vi "set_instruments (SubVI).vi"(0 "Process list":T5, 1 "Flash lamp settings:":T4={"Output channel (for flashing)"="Dev4/ao0", "Loop iteration"=0, "Path"=path "", "Flash lamp\n settings:"={"Flash lamp?"=FALSE, "Number of cyles\nbetween flashes"=3, "# Pulses"=35, "Stop flashing \nbelow thresh?"=FALSE, "Stop threshold"=0.001, "Pulse voltage?"=FALSE, "Pulse length (ms)"=0.001, "Pulse amp (V)"=0.001}}, 2 "signal type":T1(ring), 4 "electrodes reference":refnum<vi>, 5 "instrument config":T3, 6 "Num samples":i32, 7 "small amp":dbl=1.0 format="%0.2p", 9 "Volt vs pos array":cluster{dbl, dbl}[](array[cluster]), 10 "wfm?":bool, 11 "small amp freq":dbl=10.0 format="%0.2p", 12 "User Def. Wfm Name":string="RANDFREQ", 13 "Add small amp?":bool) -> (14 "Curr threshold":dbl, 18 "DC volts arr":dbl[](array[numeric]), 19 "instrum out":T2)   [LabVIEW 2014]
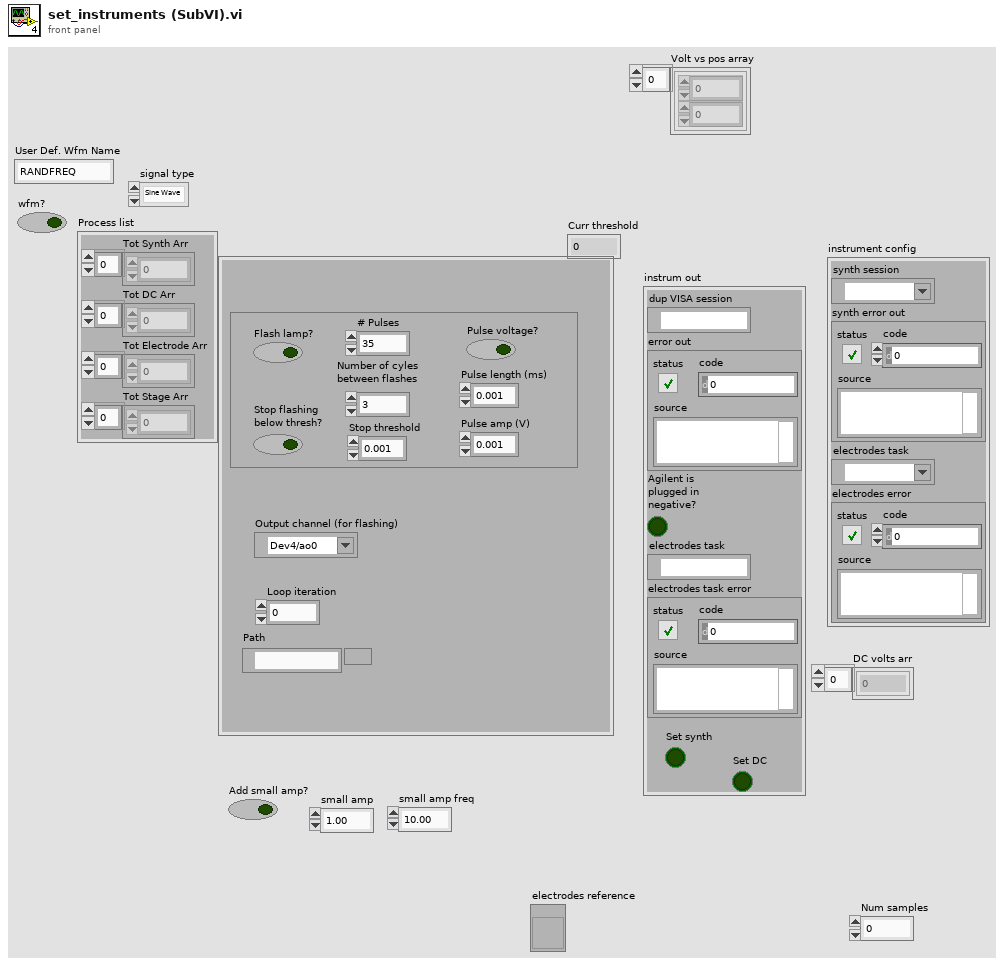
[diagram p1: front panel]
types:
  T1 = enum16{"Sine Wave", "Triangle Wave", "Square Wave", "Sawtooth Wave"}
  T2 = cluster{"dup VISA session":refnum<visa-resource-name>, "error out":errorcluster, "Agilent is \nplugged in \nnegative?":bool, "electrodes task":refnum<k21>, "electrodes task error":errorcluster, "Set synth":bool, "Set DC":bool}
  T3 = cluster{"synth session":refnum<visa-resource-name>, "synth error out":errorcluster, "electrodes task":refnum<k21>, "electrodes error":errorcluster}
  T4 = cluster{"Output channel (for flashing)":tag, "Loop iteration":i32, "Path":path, "Flash lamp\n settings:":cluster{"Flash lamp?":bool, "Number of cyles\nbetween flashes":i32, "# Pulses":i32, "Stop flashing \nbelow thresh?":bool, "Stop threshold":dbl, "Pulse voltage?":bool, "Pulse length (ms)":dbl, "Pulse amp (V)":dbl}}
  T5 = cluster{"Tot Synth Arr":dbl[], "Tot DC Arr":dbl[], "Tot Electrode Arr":dbl[], "Tot Stage Arr":dbl[]}
  T6 = cluster{"Flash lamp?":bool, "Number of cyles\nbetween flashes":i32, "# Pulses":i32, "Stop flashing \nbelow thresh?":bool, "Stop threshold":dbl, "Pulse voltage?":bool, "Pulse length (ms)":dbl, "Pulse amp (V)":dbl}
  T7 = cluster{"dup VISA session":refnum<visa-resource-name>, "error out":errorcluster, "Agilent is \nplugged in \nnegative?":bool, "electrodes task 2":refnum<k21>, "electrodes task error 2":errorcluster, "Set synth?":bool, "Set DC?":bool}
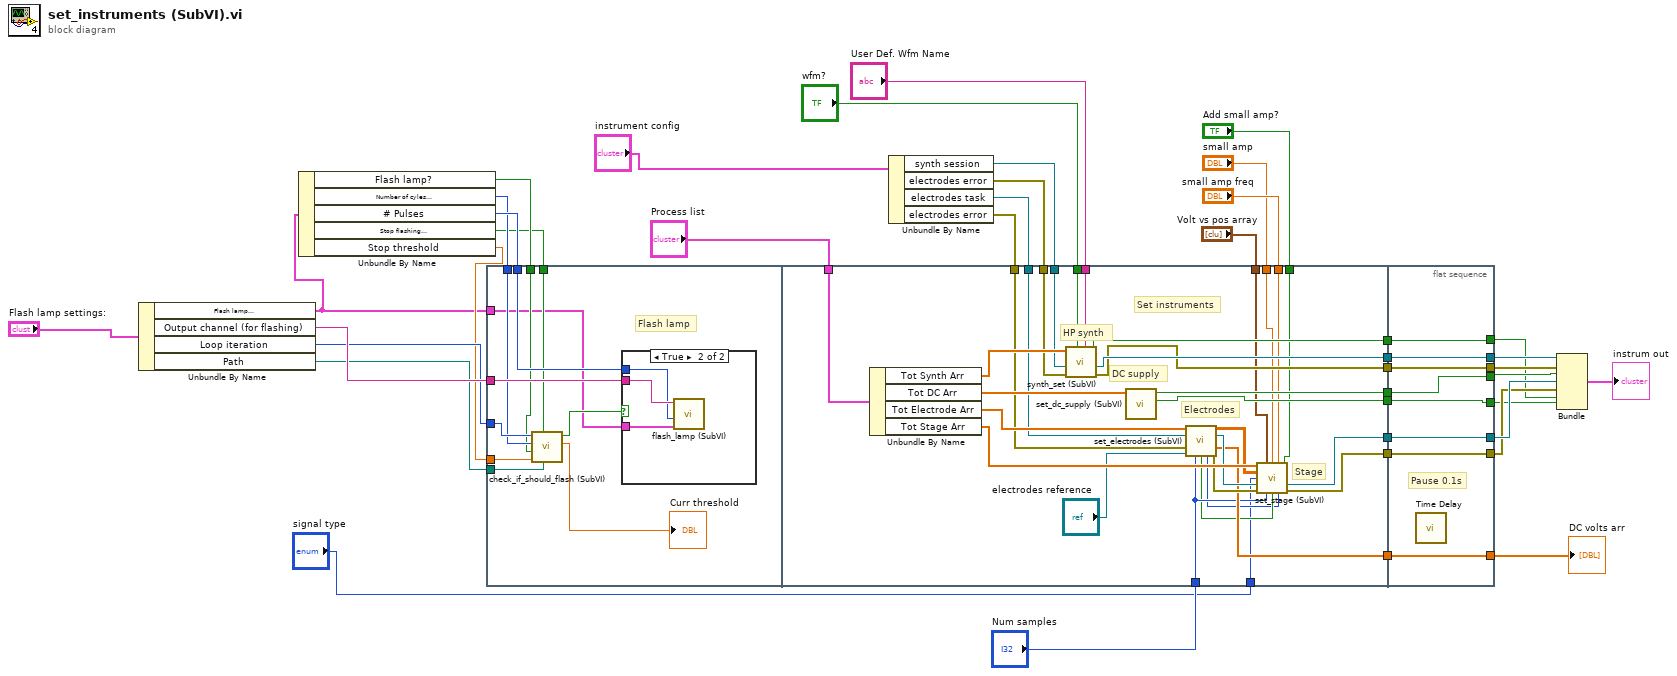
[diagram p0: block diagram]
diagram:
  n1 = Unbundle By Name("Flash lamp settings:") -> ("Flash lamp\n settings:"=w2:T6, "Output channel (for flashing)"=w39:tag, "Loop iteration"=w37:i32, "Path"=w34:path)
  n2 = Unbundle By Name(w2) -> ("Flash lamp?"=w35:bool, "Number of cyles\nbetween flashes"=w36:i32, "# Pulses"=w38:i32, "Stop flashing \nbelow thresh?"=w32:bool, "Stop threshold"=w33:dbl)
  n3 = flat-sequence {
    tunnel: w39 -> [w52]
    tunnel: w38 -> [w51]
    tunnel: w37 -> [w50]
    tunnel: w36 -> [w49]
    tunnel: w35 -> [w48]
    tunnel: w34 -> [w47]
    tunnel: w33 -> [w46]
    tunnel: w32 -> [w45]
    tunnel: w2 -> [w42]
    tunnel: "Process list" -> [w86]
    tunnel: w31 -> [w84]
    tunnel: w30 -> [w83]
    tunnel: w27 -> [w80]
    tunnel: w28 -> [w79]
    tunnel: [w69] -> w20
    tunnel: [w78] -> w19
    tunnel: [w77] -> w18
    tunnel: [w76] -> w17
    tunnel: [w68] -> w16
    tunnel: [w74] -> w15
    tunnel: [w73] -> w13
    tunnel: [w66] -> w11
    tunnel: "Num samples" -> [w65]
    tunnel: "wfm?" -> [w64]
    tunnel: "User Def. Wfm Name" -> [w63]
    tunnel: "small amp freq" -> [w60]
    tunnel: "small amp" -> [w58]
    tunnel: "Add small amp?" -> [w59]
    tunnel: "Volt vs pos array" -> [w57]
    tunnel: "signal type" -> [w56]
    tunnel: [w90] -> w22
    tunnel: [w91] -> w24
    tunnel: [w92] -> w25
    tunnel: [w93] -> w26
    tunnel: [w94] -> w23
    tunnel: w20 -> [w94]
    tunnel: w19 -> [w93]
    tunnel: w18 -> [w92]
    tunnel: w17 -> [w91]
    tunnel: w16 -> [w90]
    tunnel: w15 -> [w89]
    tunnel: [w89] -> w14
    tunnel: [w88] -> w12
    tunnel: w13 -> [w88]
    tunnel: [w87] -> w10
    tunnel: w11 -> [w87]
    frame #0 {
      # "Flash lamp"
      n4 = call "check_if_should_flash (SubVI).vi"("Path"=w47, "Stop below threshold"=w45, "Stop threshold"=w46, "Flash lamp?"=w48, "Number of cyles\nbetween flashes"=w49, "Loop iteration"=w50) -> ("Curr threshold"=→"Curr threshold":dbl, "Should flash"=w44:bool)  [unwired: 4 in]
      n5 = case shown="True" w44 {
        tunnel: w52 -> [_ w55]
        tunnel: w51 -> [_ w54]
        tunnel: w42 -> [_ w53]
        frame False {
        }
        frame True {
          n6 = call "flash_lamp (SubVI).vi"("Flash lamp\n settings:"=w53, "# Pulses in"=w54, "Output channel (for flashing)"=w55) -> ()  [unwired: 9 in]
        }
      }
    }
    frame #1 {
      # "Stage"
      # "Electrodes"
      # "DC supply"
      # "HP synth"
      # "Set instruments"
      n7 = Unbundle By Name(w86) -> ("Tot Synth Arr"=w85:dbl[], "Tot DC Arr"=w82:dbl[], "Tot Electrode Arr"=w81:dbl[], "Tot Stage Arr"=w75:dbl[])
      n8 = call "synth_set (SubVI).vi"("User Def. Wfm Name"=w63, "wfm?"=w64, "error in (no error)"=w83, "VISA session"=w84, "Tot Synth Arr"=w85) -> ("error out"=w77:errorcluster, "dup VISA session"=w78:refnum<visa-resource-name>, "Set synth?"=w73:bool)  [unwired: 4 in]
      n9 = call "set_dc_supply (SubVI).vi"("Tot DC Arr"=w82) -> ("Set DC?"=w74:bool, "Agilent is \nplugged in \nnegative?"=w76:bool)  [unwired: 9 in]
      n10 = call "set_electrodes (SubVI).vi"("Tot Electrode Arr"=w81, "electrodes task 2"=w80, "electrodes error"=w79, "electrodes reference"="electrodes reference", "Num samples"=w65) -> ("electrode arr"=w72:dbl[][], "electrodes task"=w71:refnum<k21>, "DC volts arr"=w66:dbl[], "Use arbitrary\nforce func?"=w62:bool, "Electrode to sweep:"=w61:i32, "electrodes task error"=w70:errorcluster)  [unwired: 5 in]
      n11 = call "set_stage (SubVI).vi"("Tot Stage Arr"=w75, "Volt vs pos array"=w57, "small amp"=w58, "small amp freq"=w60, "Add small amp?"=w59, "electrode arr"=w72, "signal type"=w56, "electrodes task"=w71, "electrodes task error"=w70, "Num samples"=w65, "Use arb force?"=w62, "Electrode to sweep"=w61) -> ("electrodes task 2"=w69:refnum<k21>, "electrodes task error 2"=w68:errorcluster)  [unwired: 2 in]
    }
    frame #2 {
      # "Pause 0.1s"
      n12 = call "Time Delay"() -> ()  [unwired: 11 in, 1 out]
    }
  }
  n13 = Unbundle By Name("instrument config") -> ("synth session"=w31:refnum<visa-resource-name>, "electrodes error"=w30:errorcluster, "electrodes task"=w27:refnum<k21>, "electrodes error"=w28:errorcluster)
  n14 = Bundle("dup VISA session"=w26, "error out"=w25, "Agilent is \nplugged in \nnegative?"=w24, "electrodes task 2"=w23, "electrodes task error 2"=w22, "Set synth?"=w12, "Set DC?"=w14) -> (→"instrum out":T7)  [unwired: 1 in]
  "DC volts arr" <- w10
